vi "Quadratic_Equation_Calc.vi"() -> ()   [LabVIEW 2025]
panel:
  out "X2":dbl
  out "X1":dbl
  in  "c":dbl
  in  "b":dbl
  in  "a":dbl
  # "X"
  # "+"
  # "X"
  # "2"
  # "+"
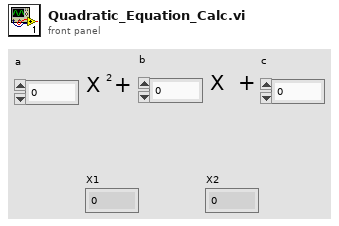
[diagram p1: front panel]
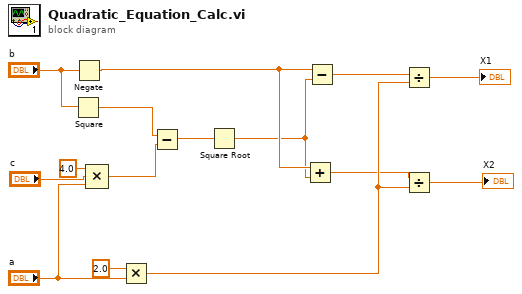
[diagram p0: block diagram]
diagram:
  n1 = Square(x="b") -> (x^2=w8:dbl)
  n2 = Negate(x="b") -> (-x=w10:dbl)
  n3 = Compound Arithmetic op=MULTIPLY(4.0 ("value"), "c", "a") -> (w4:dbl)
  n4 = Multiply(x=2.0, y="a") -> (x*y=w12:dbl)
  n5 = Subtract(x=w8, y=w4) -> (x-y=w3:dbl)
  n6 = Square Root(x=w3) -> (sqrt(x)=w2:dbl)
  n7 = Add(x=w10, y=w2) -> (x+y=w1:dbl)
  n8 = Subtract(x=w10, y=w2) -> (x-y=w11:dbl)
  n9 = Divide(x=w11, y=w12) -> (x/y=→"X1":dbl)
  n10 = Divide(x=w1, y=w12) -> (x/y=→"X2":dbl)
